vi "Test Probe on Wire Exists - with probes.vi"() -> (0 "error out":errorcluster)   [LabVIEW 2020]
doc: "Test of <b>Probe on Wire Exists.vi</b>: check that the VI detects probes."
uses:
  <vilib>/addons/_JKI Toolkits/Caraya/classes/Test/Test.lvclass
  <vilib>/addons/_JKI Toolkits/Caraya/classes/Assert/Assert.lvclass
  src/Type Definitions/Class Name--enum.ctl
  <vilib>/Utility/traverseref.llb/VI Scripting - Traverse.lvlib
  <vilib>/Utility/traverseref.llb/TRef TravTarget.ctl
  <vilib>/addons/_JKI Toolkits/Caraya/classes/Assert/Assert True.vi
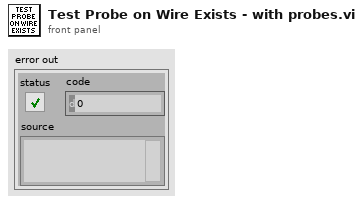
[diagram p1: front panel]
types:
  T1 = typedef "Class Name--enum.ctl" = enum16{"Node", "Wire"}
  T2 = typedef "TRef TravTarget.ctl" = enum16{"FP", "BD", "Other"}
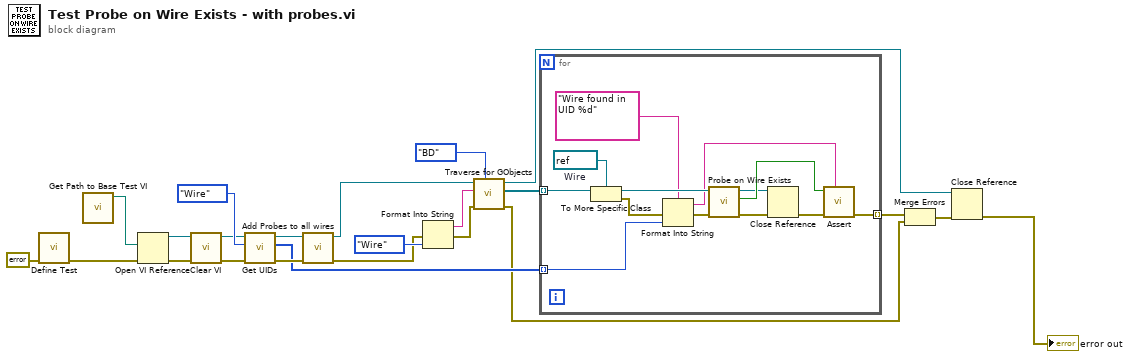
[diagram p0: block diagram]
diagram:
  n1 = call <vilib>:"Define Test.vi"("error in (no error)"=errorcluster {"status"=FALSE, "code"=0, "source"=""}) -> ("error out"=w4:errorcluster)  [unwired: 9 in, 1 out]
  n2 = call "Get Path to Base Test VI.vi"() -> ("Path"=w12:path)  [unwired: 11 in]
  n3 = Open VI Reference(vi path=w12, error in (no error)=w4) -> (vi reference=w2:refnum<vi>, error out=w7:errorcluster)  [unwired: 4 in]
  n4 = call "Clear VI.vi"("error in"=w7, "VI Refnum In"=w2) -> ("error out"=w3:errorcluster, "VI Refnum Out"=w1:refnum<vi>)  [unwired: 8 in]
  n5 = call "Get UIDs.vi"("error in"=w3, "Class Name"=Class_Name--enum."Wire", "VI Refnum In"=w1) -> ("error out"=w15:errorcluster, "UIDs"=w9:i32[], "VI Refnum Out"=w10:refnum<vi>)  [unwired: 6 in]
  n6 = call "Add Probes to all wires.vi"("error in"=w15, "VI Refnum In"=w10) -> ("error out"=w14:errorcluster, "VI Refnum Out"=w13:refnum<vi>)  [unwired: 8 in]
  n7 = Format Into String(error in=w14, Class_Name--enum."Wire" ("Class Name")) -> (resulting string=w20:string, error out=w19:errorcluster)  [unwired: 2 in]
  n8 = call <vilib>:"Traverse for GObjects.vi"("Traverse Target"=TRef_TravTarget."BD", "error in (no error)"=w19, "Class Name"=w20, "VI Refnum"=w13) -> ("error out"=w8:errorcluster, "References"=w18:refnum<vi>[], "dup VI Refnum"=w6:refnum<vi>)  [unwired: 4 in, 1 out]
  n9 = for {
    tunnel: w18 -> [w36] mode=indexing
    tunnel: w9 -> [w31] mode=indexing
    tunnel: [w27] -> w17 mode=indexing
    w35 = refnum<vi> refnum  # Wire
    n10 = To More Specific Class(target class=w35, reference=w36) -> (specific class reference=w34:refnum<vi>, error out=w30:errorcluster)  [unwired: 1 in]
    n11 = Format Into String(format string="Wire found in UID %d", error in=w30, w31) -> (resulting string=w28:string, error out=w29:errorcluster)  [unwired: 1 in]
    n12 = call "Probe on Wire Exists.vi"("error in"=w29, "Wire in"=w34) -> ("error out"=w25:errorcluster, "Probe Exists"=w33:bool, "Wire out"=w26:refnum<vi>)  [unwired: 6 in, 1 out]
    n13 = Close Reference(reference=w26, error in (no error)=w25) -> (error out=w24:errorcluster)
    n14 = call-poly <vilib>:"Assert.vi"("Label"=w28, "error in (no error)"=w24, "True?"=w33) -> ("error out"=w27:errorcluster)  [unwired: 7 in, 1 out]
  }
  n15 = Merge Errors(w17, w8) -> (w5:errorcluster)
  n16 = Close Reference(reference=w6, error in (no error)=w5) -> (error out=→"error out":errorcluster)
